vi "SaveControlValues.vi"(8 "error in":errorcluster, 11 "ControlValues in":refnum<class "ControlValues.lvclass">) -> (0 "error out":errorcluster, 3 "ControlValues out":refnum<class "ControlValues.lvclass">, 5 "Debug":string)   [LabVIEW 2014, in "ControlValues.lvclass"]
uses:
  ControlValues.lvclass
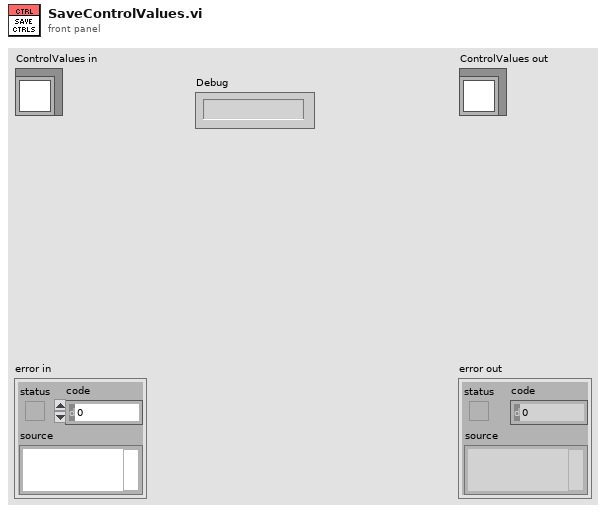
[diagram p1: front panel]
types:
  T1 = enum32{"invalid app kind", "Development System", "Run Time System", "Student Edition", "Embedded LabVIEW", "Evaluation", "Custom"}
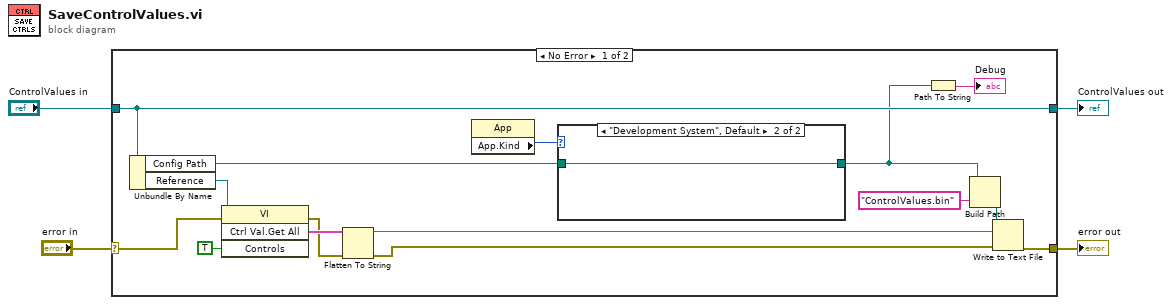
[diagram p0: block diagram]
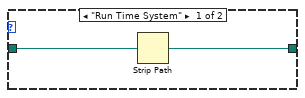
[diagram p2: hidden frame]
diagram:
  n1 = case shown="No Error" "error in" {
    selector: "error in" -> [w12 w24]
    tunnel: [w10 w24] -> w3
    tunnel: [w15 w23] -> w1
    tunnel: "ControlValues in" -> [w15 w23]
    frame No Error {
      n2 = Unbundle By Name(w15) -> ("Config Path"=w6:path, "Reference"=w14:refnum<vi>)
      n3 = invoke class="VI" method="Ctrl Val.Get All"(reference=w14, error in=w12, "Controls"=TRUE) -> (error out=w11:errorcluster, "Get All Control Values Variant"=w18:cluster{"Name":string, "Variant Data":variant}[])  [unwired: 1 in, 2 out]
      n4 = Flatten To String(anything=w18, error in (no error)=w11) -> (data string=w17:string, error out=w7:errorcluster)  [unwired: 2 in, 1 out]
      n5 = property class="App"() -> ("App.Kind"=w8:T1)  [unwired: 2 in, 2 out]
      n6 = case shown="\"Development System\", Default" w8 {
        tunnel: [w20 w22] -> w5
        tunnel: w6 -> [w21 w22]
        frame "Run Time System" {
          n7 = Strip Path(path=w21) -> (stripped path=w20:path)  [unwired: 1 out]
        }
        frame "Development System", Default {
        }
      }
      n8 = Path To String(path=w5) -> (string=→"Debug":string)
      n9 = Build Path(base path=w5, name or relative path="ControlValues.bin") -> (appended path=w13:path)
      n10 = Write to Text File(file (use dialog)=w13, text=w17, error in=w7) -> (error out=w10:errorcluster)  [unwired: 1 in, 2 out]
    }
    frame Error {
    }
  }
  "error out" <- w3
  "ControlValues out" <- w1
